vi "LastStepMsgParser.vi"(7 "Out MSG Names":string[](array[string]), 9 "Out MSG Codes":string[](array[string]), 10 "Msg Array":T1(array[cluster])) -> (0 "Output Alg Msg":string[][](table), 2 "code":i32[](array[numeric]), 3 "current msg num":i32)   [LabVIEW 2010]
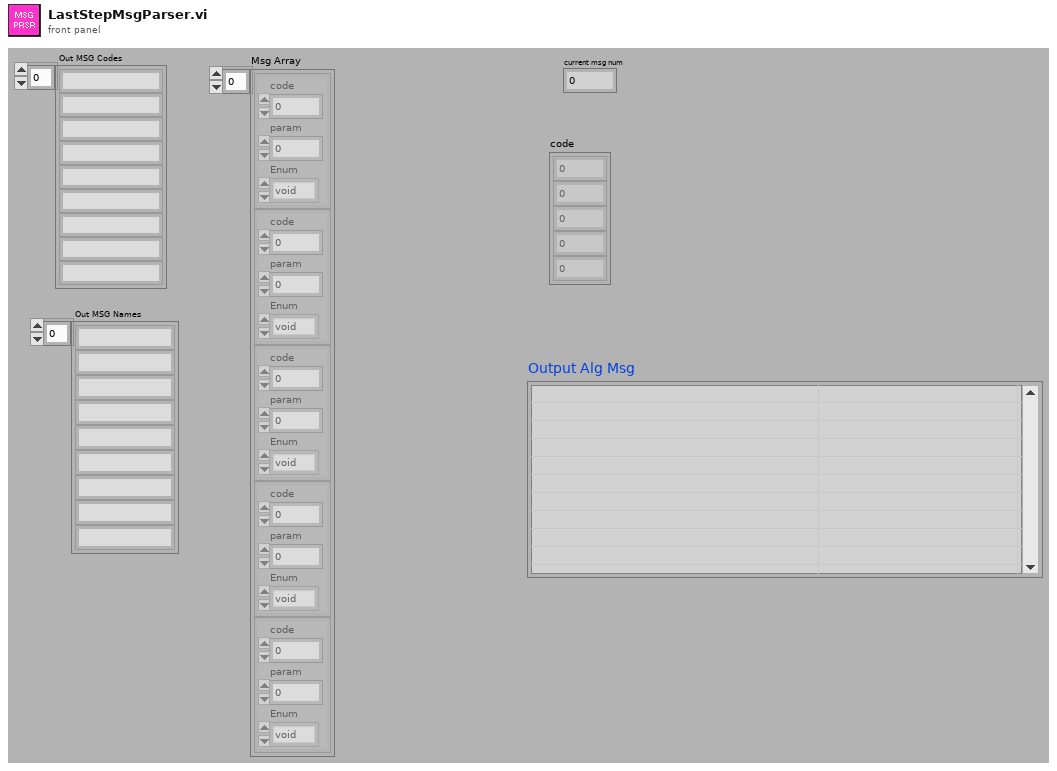
[diagram p1: front panel]
types:
  T1 = cluster{"code":i32, "param":i32, "Enum":enum16{"void", "byte", "int", "float"}}[]
  T2 = cluster{"code":i32, "param":i32, "Enum":enum16{"void", "byte", "int", "float"}}
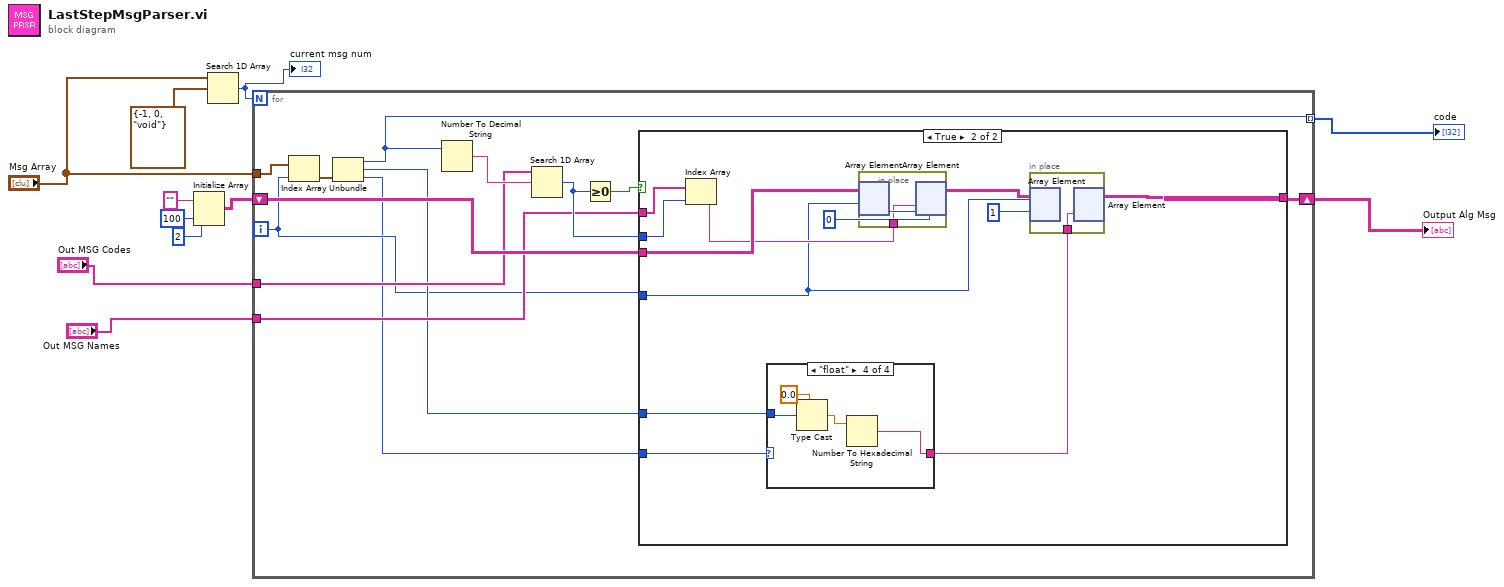
[diagram p0: block diagram]
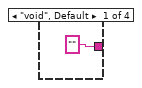
[diagram p3: hidden frame]
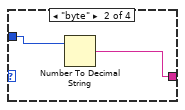
[diagram p4: hidden frame]
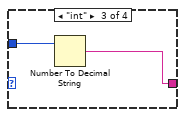
[diagram p5: hidden frame]
diagram:
  n1 = Initialize Array("", 100 ("dimension size"), 2 ("dimension size")) -> (w1:string[][])
  n2 = Search 1D Array(1D array="Msg Array", element=T2 {"code"=-1, "param"=0, "Enum"=enum."void"} ("Cluster")) -> (index of element=w5:i32)  [unwired: 1 in]
  "current msg num" <- w5
  n3 = for {
    N: w5 -> [_]
    tunnel: "Msg Array" -> [w15]
    tunnel: [w24] -> w9 mode=indexing
    shift-right: [w19] -> w8
    shift-left: w1 -> [w20]
    tunnel: "Out MSG Codes" -> [w18]
    tunnel: "Out MSG Names" -> [w17]
    i -> [w14]
    n4 = Index Array(array=w15, index=w14) -> (element=w13:T2)
    n5 = Unbundle(w13) -> ("code"=w24:i32, "param"=w16:i32, "Enum"=w12:enum16{"void", "byte", "int", "float"})
    n6 = Number To Decimal String(number=w24) -> (decimal integer string=w23:string)  [unwired: 1 in]
    n7 = Search 1D Array(1D array=w18, element=w23) -> (index of element=w21:i32)  [unwired: 1 in]
    n8 = Greater Or Equal To 0?(x=w21) -> (x >= 0?=w22:bool)
    n9 = case shown="True" w22 {
      tunnel: w17 -> [_ w37]
      tunnel: w21 -> [_ w36]
      tunnel: w16 -> [_ w28]
      tunnel: w20 -> [w25 w31]
      tunnel: [w25 w32] -> w19
      tunnel: w14 -> [_ w26]
      tunnel: w12 -> [_ w29]
      frame False {
      }
      frame True {
        n10 = Index Array(array=w37, index=w36) -> (element=w30:string)
        n11 = case shown="\"float\"" w29 {
          tunnel: w28 -> [_ w40 w42 w46]
          tunnel: ["" ("decimal integer string") w39 w41 w43] -> w27
          frame "void", Default {
          }
          frame "byte" {
            n12 = Number To Decimal String(number=w40) -> (decimal integer string=w39:string)  [unwired: 1 in]
          }
          frame "int" {
            n13 = Number To Decimal String(number=w42) -> (decimal integer string=w41:string)  [unwired: 1 in]
          }
          frame "float" {
            n14 = Type Cast(type=0.0 ("default (0 dbl)"), x=w46) -> (*(type *) &x=w44:dbl)
            n15 = Number To Hexadecimal String(2:w44) -> (0:w43:string)  [unwired: 1 in]
          }
        }
        n16 = in-place {
          in-place-border: w30 -> [w48]
          n17 = in-place-array #1(w31, w26, 0) -> ()  [unwired: 1 out]
          n18 = in-place-array #1(w48) -> (w34:string[][])  [unwired: 2 out]
        }
        n19 = in-place {
          in-place-border: w27 -> [w47]
          n20 = in-place-array #2(w34, w26, 1) -> ()  [unwired: 1 out]
          n21 = in-place-array #2(w47) -> (w32:string[][])  [unwired: 2 out]
        }
      }
    }
  }
  "code" <- w9
  "Output Alg Msg" <- w8
